vi "FPGA Target Approach Retraction2 (1).vi"() -> ()   [LabVIEW 2013]
uses:
  <vilib>/eio/EIONode/EIONode.xnode
  <vilib>/rvi/eio/common/nirviEmuTemplateMethod_errors.vi
panel:
  in  "Automated FPGA Start":bool
  out "Counter Output 2":dbl
  in  "Approach Speed (nm/s)":dbl=5.0
  in  "Bit/nm converter":dbl=0.9155413
  out "Bit/ms":dbl
  out "Multiplier":dbl format="%#_13g"
  out "Numeric 3":dbl format="%#_13g"
  out "Numeric":dbl format="%#_13g"
  in  "Manual FPGA Start":bool
  out "FPGA Output Voltage":fxp<+/-,64,32>
  out "Z Fine Indicator":fxp<+/-,40,30>
  out "Counter Indicator":i32
  in  "Z Fine Output":fxp<+/-,40,30>
  in  "Counter Output":i32
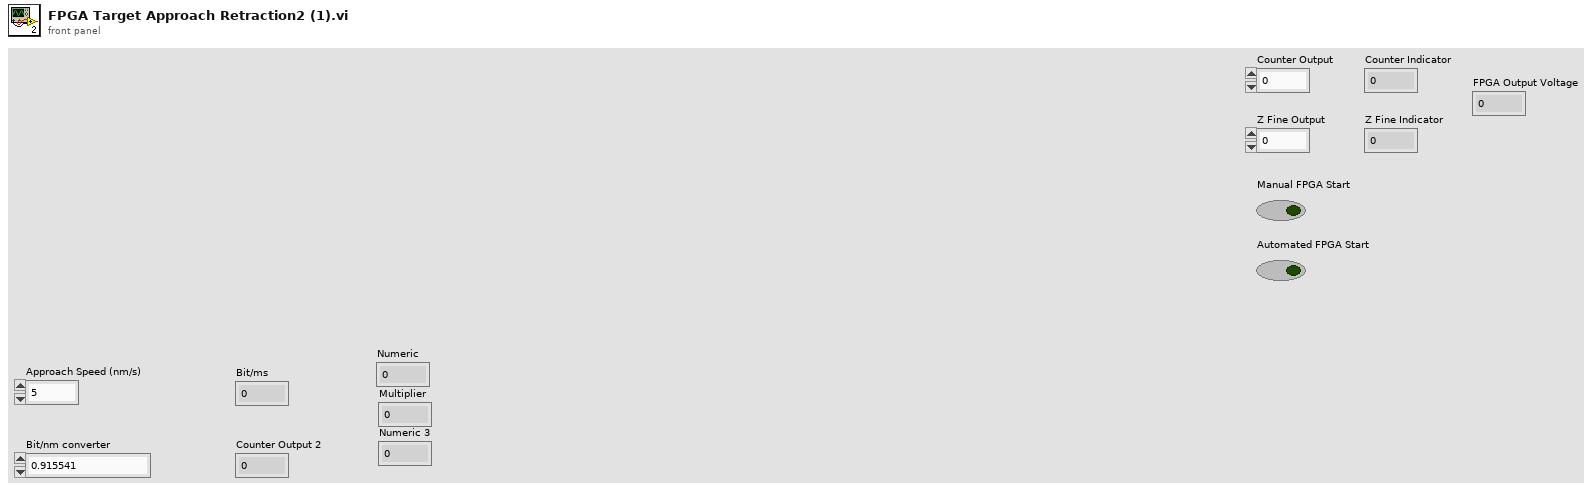
[diagram p1: front panel]
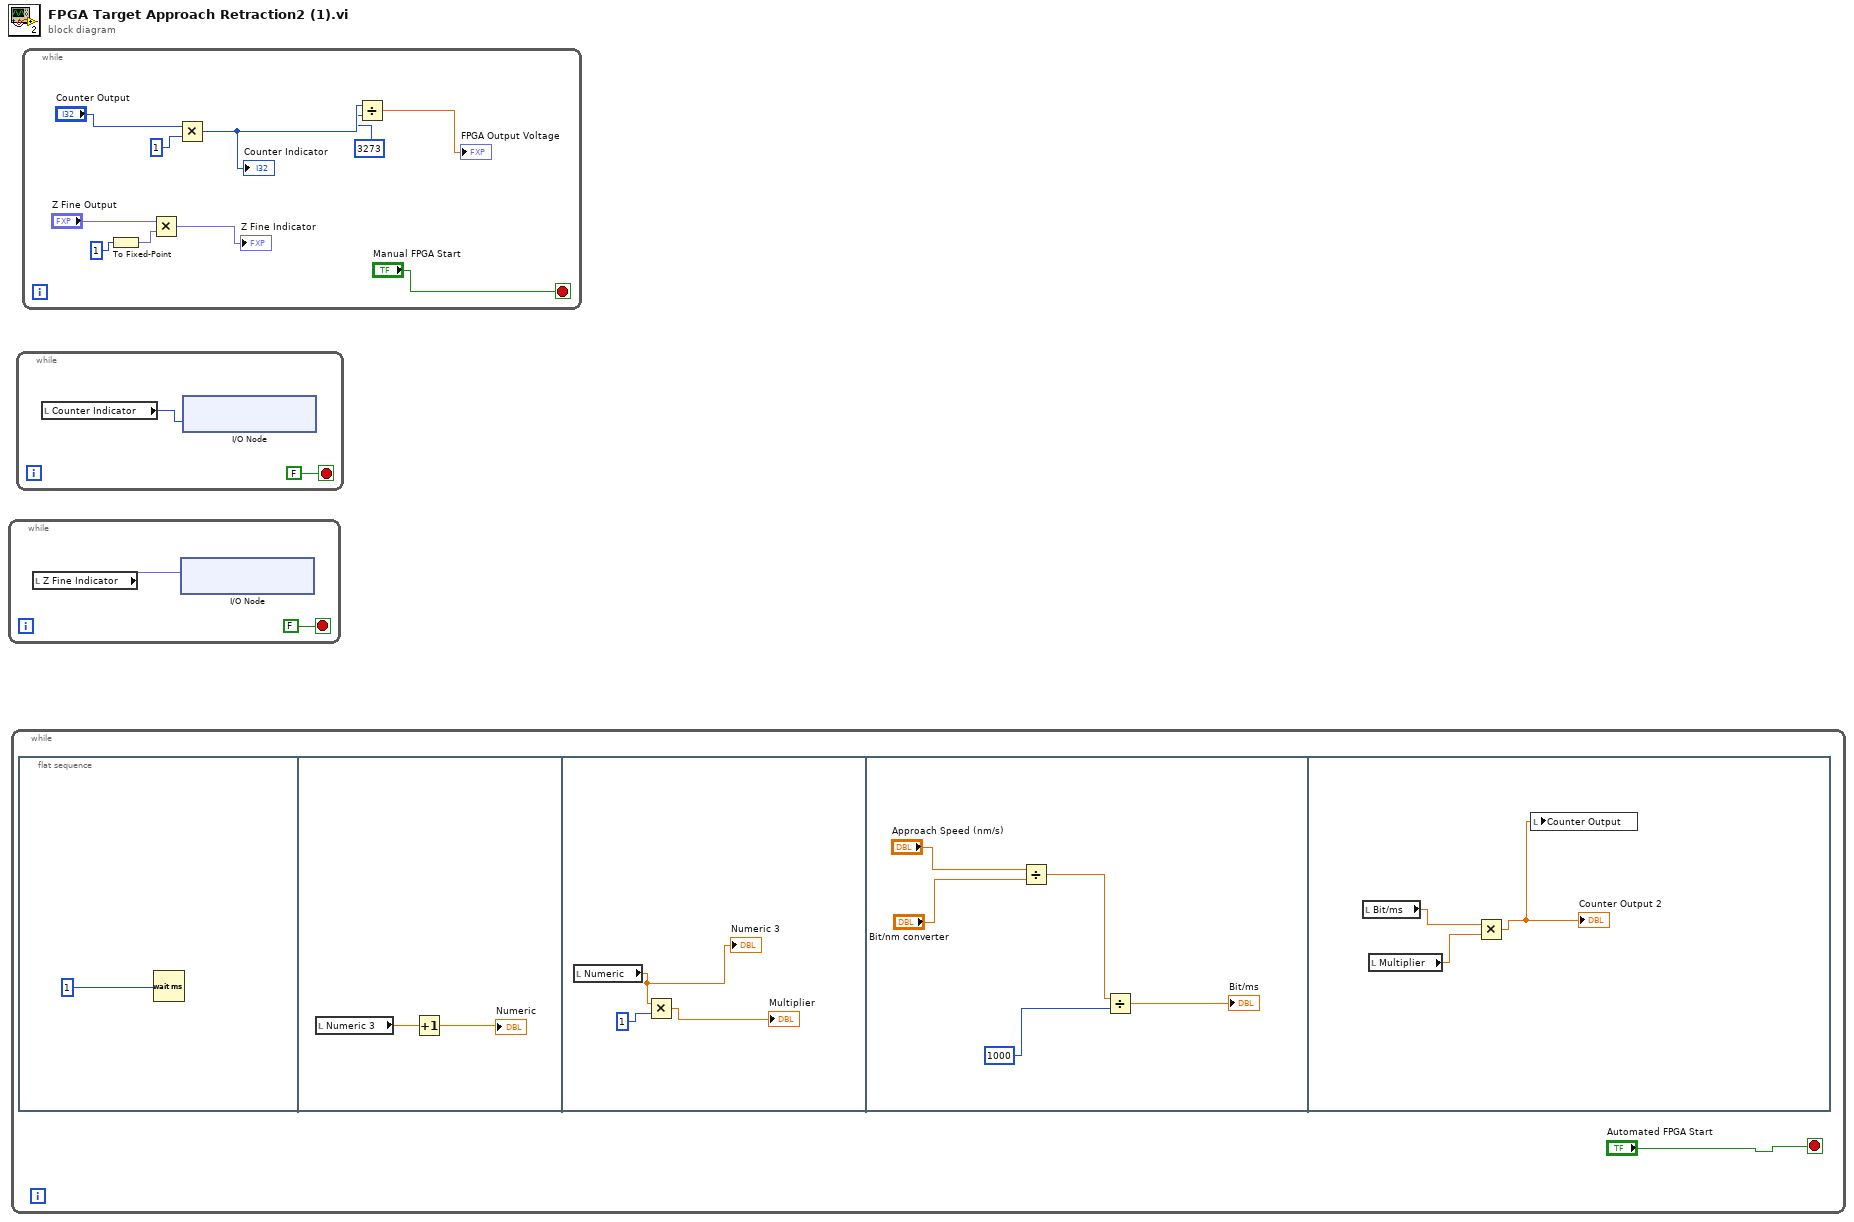
[diagram p0: block diagram]
diagram:
  n1 = while {
    stop <- FALSE stop-if-true
    n2 = local read "Z Fine Indicator"() -> (w1:fxp<+/-,40,30>)
    n3 = xnode "I/O Node"("Connector0/AO2"=w1) -> ()  [unwired: 1 in, 1 out]
  }
  n4 = while {
    stop <- "Automated FPGA Start" stop-if-true
    n5 = flat-sequence {
      frame #0 {
        n6 = Wait (ms)(milliseconds to wait=1) -> ()  [unwired: 1 out]
      }
      frame #1 {
        n7 = local read "Numeric 3"() -> (w6:dbl)
        n8 = Increment(x=w6) -> (x+1=→"Numeric":dbl)
      }
      frame #2 {
        n9 = local read "Numeric"() -> (w7:dbl)
        "Numeric 3" <- w7
        n10 = Multiply(x=w7, y=1) -> (x*y=→"Multiplier":dbl)
      }
      frame #3 {
        n11 = Divide(x="Approach Speed (nm/s)", y="Bit/nm converter") -> (x/y=w10:dbl)
        n12 = Divide(x=w10, y=1000) -> (x/y=→"Bit/ms":dbl)
      }
      frame #4 {
        n13 = local read "Bit/ms"() -> (w16:dbl)
        n14 = local read "Multiplier"() -> (w17:dbl)
        n15 = Multiply(x=w16, y=w17) -> (x*y=w15:dbl)
        "Counter Output 2" <- w15
        n16 = local write "Counter Output"(w15) -> ()
      }
    }
  }
  n17 = while {
    stop <- FALSE stop-if-true
    n18 = local read "Counter Indicator"() -> (w18:i32)
    n19 = xnode "I/O Node"("Connector0/AO7"=w18) -> ()  [unwired: 1 in, 1 out]
  }
  n20 = while {
    stop <- "Manual FPGA Start" stop-if-true
    n21 = To Fixed-Point(number=1) -> (fixed-point=w25:fxp<+/-,32,32>)  [unwired: 1 in]
    n22 = Multiply(x="Z Fine Output", y=w25) -> (x*y=→"Z Fine Indicator":fxp<+/-,64,62>)
    n23 = Multiply(x="Counter Output", y=1) -> (x*y=w24:i32)
    "Counter Indicator" <- w24
    n24 = Divide(x=w24, y=3273) -> (x/y=→"FPGA Output Voltage":dbl)
  }
